vi "HMI.vi"(8 "error in (no error)":errorcluster caption="entrée d'erreur (pas d'erreur)", 11 "Popup Operator_Input Batch In":refnum<class "Class Popup Operator_Input Batch.lvclass">) -> (0 "error out":errorcluster caption="sortie d'erreur", 1 "Input":string="Attente \nvalidation", 2 "Operator_Selection":bool, 3 "Popup Operator_Input Batch In":refnum<class "Class Popup Operator_Input Batch.lvclass">)   [LabVIEW 2020, in "Library Instrument & Equipement.lvlib" / "Library Popup.lvlib" / "Class Popup Operator_Input Batch.lvclass"]
uses:
  Class Popup Operator_Input Batch.lvclass
  C:/Users/ngarcin/OneDrive - Altyor/Standard TB/Class/Popup/Class Popup (Main)/Class Popup (Main).lvclass
  Class Popup (Main)/Class Popup (Main).lvclass
  Class Popup Operator_Input Batch.lvclass/Class Popup Operator_Input Batch.ctl
panel:
  in  "Bouton NOK":bool
  in  "Input OP":string="Attente \nvalidation"
  in  "Bouton OK":bool
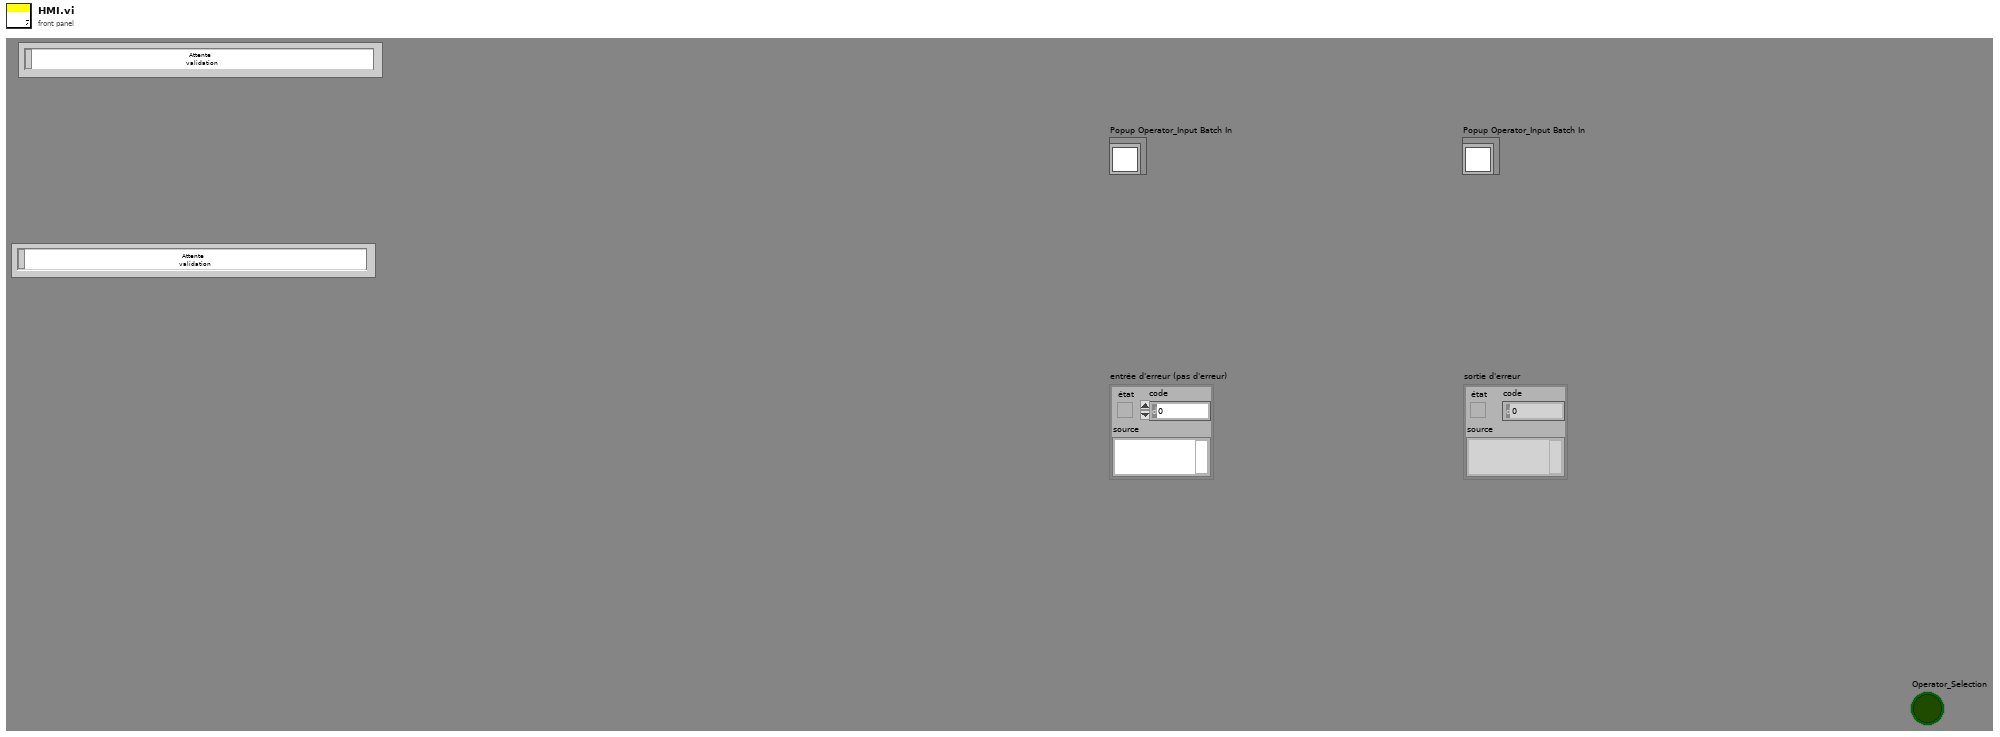
[diagram p1: front panel]
types:
  T1 = enum32{"Invalid", "Standard", "Closed", "Hidden", "Minimized", "Maximized"}
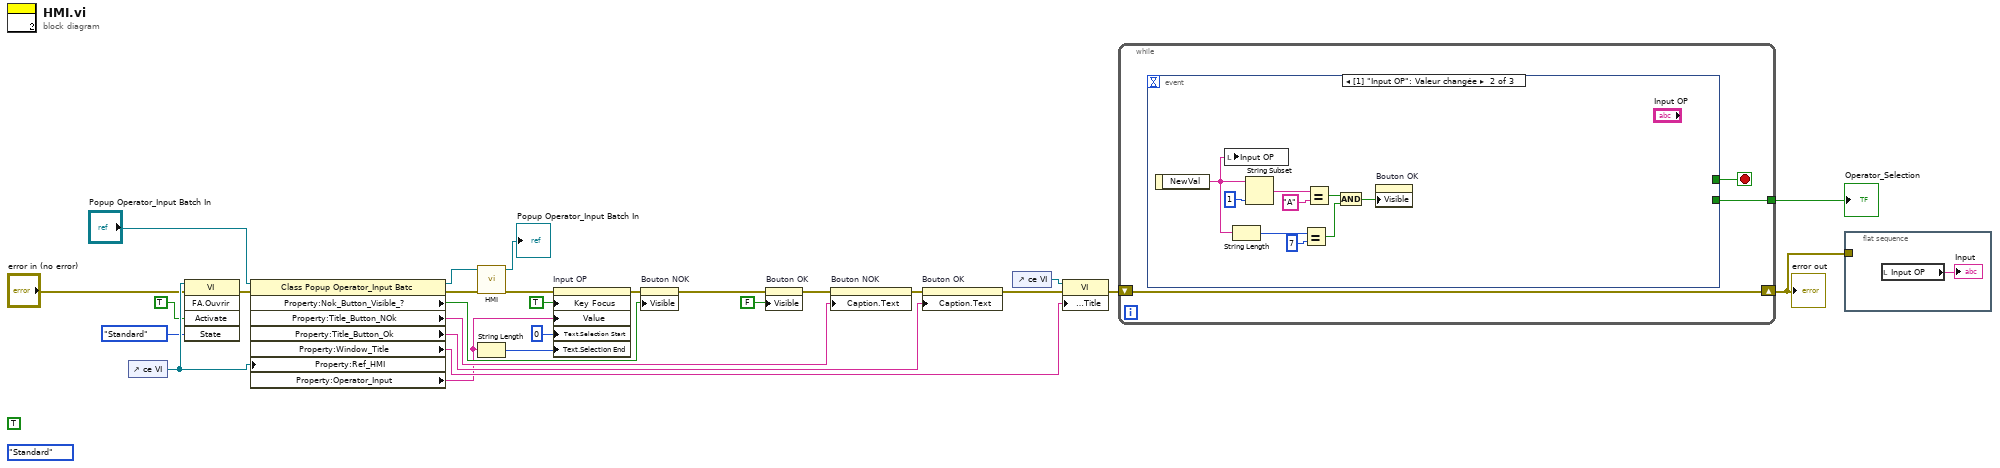
[diagram p0: block diagram]
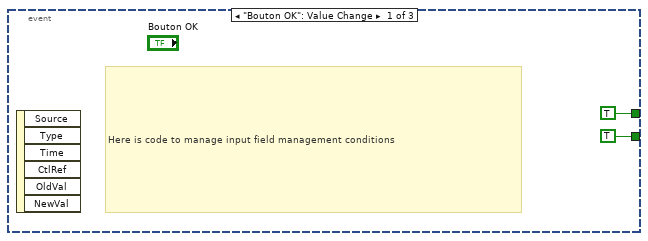
[diagram p2: hidden frame]
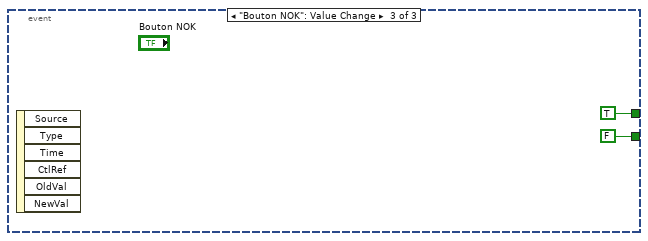
[diagram p3: hidden frame]
diagram:
  (unwired) T1."Standard" ("État")
  (unwired) TRUE ("Activer ?")
  n1 = control-ref of="ce VI"() -> (w8:refnum<vi>)
  n2 = invoke class="VI" method="FA.Ouvrir"(reference=w8, error in="error in (no error)", "Activate"=TRUE ("Activer ?"), "State"=T1."Standard" ("État")) -> (error out=w5:errorcluster)  [unwired: 1 in, 4 out]
  n3 = property class="Class Popup Operator_Input Batc"(reference="Popup Operator_Input Batch In", error in=w5, "Property:Ref_HMI"=w8) -> (reference out=w23:refnum<class "Class Popup Operator_Input Batch.lvclass">, error out=w3:errorcluster, "Property:Nok_Button_Visible_?"=w28:bool, "Property:Title_Button_NOk"=w22:string, "Property:Title_Button_Ok"=w20:string, "Property:Window_Title"=w25:string, "Property:Operator_Input"=w12:string)
  n4 = call-parent "HMI.vi"("error in (no error)"=w3, "Class Popup (Main) en entrée"=w23) -> ("error out"=w2:errorcluster, "Class Popup (Main) en sortie"=→"Popup Operator_Input Batch In":refnum<class "Class Popup Operator_Input Batch.lvclass">)  [unwired: 6 in, 2 out]
  n5 = String Length(string=w12) -> (length=w14:i32)
  n6 = property on="Input OP" class="Ch"(error in=w2, "Key Focus"=TRUE ("Focus clavier"), "Value"=w12, "Text.Selection Start"=u32 0 ("Texte.Sélection:Début"), "Text.Selection End"=w14) -> (error out=w1:errorcluster)  [unwired: 1 in, 1 out]
  n7 = property on="Bouton NOK" class="Bool"(error in=w1, "Visible"=w28) -> (error out=w18:errorcluster)  [unwired: 1 in, 1 out]
  n8 = property on="Bouton OK" class="Bool"(error in=w18, "Visible"=FALSE ("Activer ?")) -> (error out=w17:errorcluster)  [unwired: 1 in, 1 out]
  n9 = property on="Bouton NOK" class="Bool"(error in=w17, "Caption.Text"=w22) -> (error out=w21:errorcluster)  [unwired: 1 in, 1 out]
  n10 = property on="Bouton OK" class="Bool"(error in=w21, "Caption.Text"=w20) -> (error out=w15:errorcluster)  [unwired: 1 in, 1 out]
  n11 = control-ref of="ce VI"() -> (w26:refnum<vi>)
  n12 = property class="VI"(reference=w26, error in=w15, "Front Panel.Title"=w25) -> (error out=w24:errorcluster)  [unwired: 1 out]
  n13 = while {
    tunnel: [w29] -> w27
    shift-right: [w30] -> w11
    shift-left: w24 -> [w30]
    stop <- w31 stop-if-true
    n14 = event shown="[1] \"Input OP\": Valeur changée" {
      selector: _ -> [_ _ _]
      dyn-events: _ -> [_ _ _]
      timeout: _ -> [_ _ _]
      tunnel: [TRUE ("Valeur (Signalisation)") _ TRUE ("Valeur (Signalisation)")] -> w31
      tunnel: [TRUE ("Operator_Selection") _ FALSE ("Operator_Selection")] -> w29
      event "Bouton OK": Value Change {
        # "Here is code to manage input field management conditions"
        n15 = event-data() -> ()  [unwired: 1 in, 6 out]
      }
      event "Input OP": Value Change {
        n16 = event-data() -> ("NewVal"=w34:string)  [unwired: 1 in]
        n17 = local write "Input OP"(w34) -> ()
        n18 = String Length(string=w34) -> (length=w38:i32)
        n19 = String Subset(string=w34, length (rest)=1 ("longueur (reste)")) -> (substring=w41:string)  [unwired: 1 in]
        n20 = Equal?(x=w38, y=7) -> (x = y?=w36:bool)
        n21 = Equal?(x=w41, y="A") -> (x = y?=w39:bool)
        n22 = And(x=w39, y=w36) -> (x .and. y?=w35:bool)
        n23 = property on="Bouton OK" class="Bool"("Visible"=w35) -> ()  [unwired: 2 in, 2 out]
      }
      event "Bouton NOK": Value Change {
        n24 = event-data() -> ()  [unwired: 1 in, 6 out]
      }
    }
  }
  "error out" <- w11
  "Operator_Selection" <- w27
  n25 = flat-sequence {
    tunnel: w11 -> [_]
    frame #0 {
      n26 = local read "Input OP"() -> (→"Input":string)
    }
  }
